vi "Files.Get Result Dir List from Root Dir.vi"(10 "SN Len":i32=10, 11 "RootDir":path) -> (2 "Cnt":i32, 3 "Result Dirs":path[](array[path]))   [LabVIEW 2024]
panel:
  # "Result = SN_Date_Time. . . .\nEX: FB94414A63_20191118_103814"
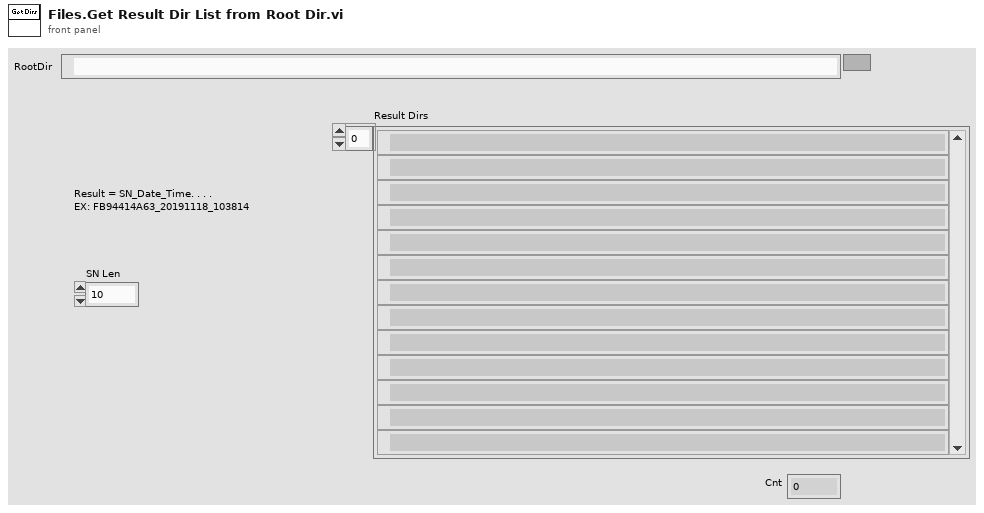
[diagram p1: front panel]
types:
  T1 = cluster{"RsltDirs":path[], "RootDir":path, "RootName":string}
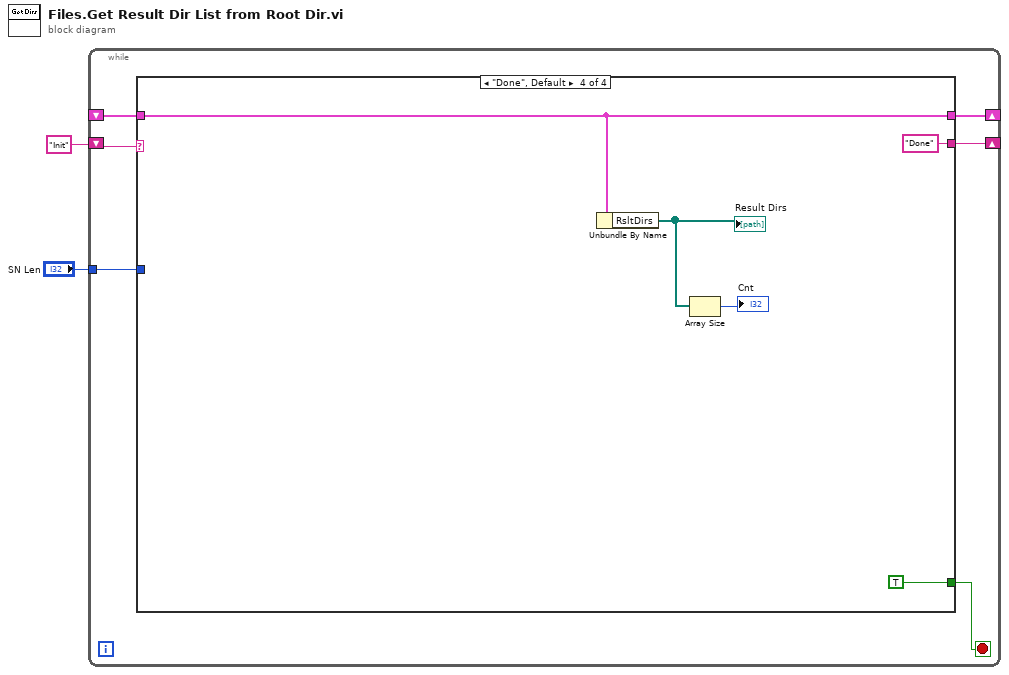
[diagram p0: block diagram]
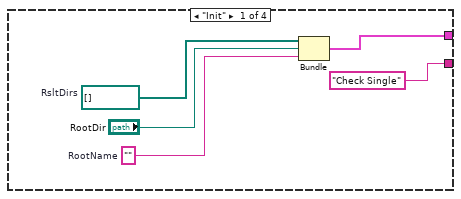
[diagram p2: hidden frame]
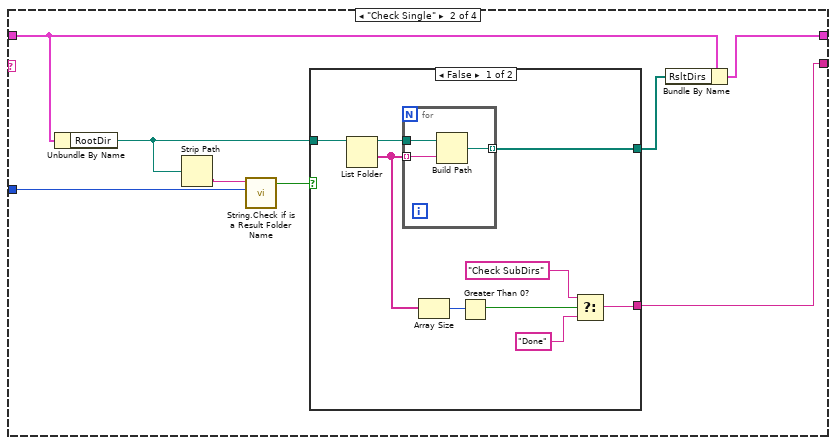
[diagram p3: hidden frame]
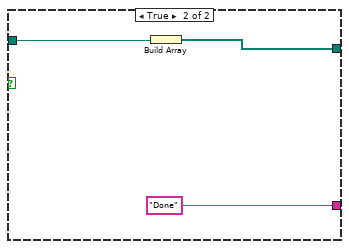
[diagram p4: hidden frame]
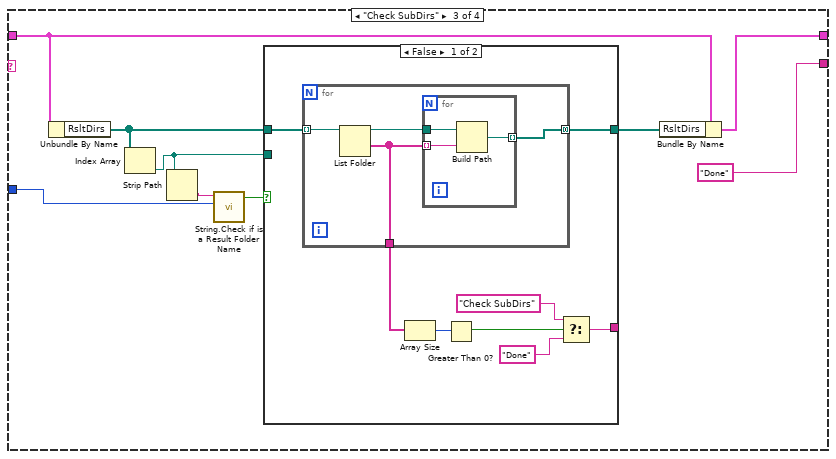
[diagram p5: hidden frame]
diagram:
  n1 = while {
    shift-right: [w6] -> _
    shift-left: _ -> [w7]
    shift-right: [w5] -> _
    shift-left: "Init" -> [w8]
    tunnel: "SN Len" -> [w3]
    stop <- w4 stop-if-true
    n2 = case shown="\"Done\", Default" w8 {
      tunnel: w7 -> [_ w20 w44 w64]
      tunnel: [w12 w21 w45 w64] -> w6
      tunnel: ["Check Single" w15 "Done" "Done"] -> w5
      tunnel: [_ _ _ TRUE] -> w4
      tunnel: w3 -> [_ w18 w40 _]
      frame "Init" {
        w10 = ""  # RootName
        w13 = path[] []  # RsltDirs
        n3 = Bundle("RsltDirs"=w13, "RootDir"="RootDir", "RootName"=w10) -> (w12:T1)  [unwired: 1 in]
      }
      frame "Check Single" {
        n4 = Unbundle By Name(w20) -> ("RootDir"=w16:path)
        n5 = Strip Path(path=w16) -> (name=w19:string)  [unwired: 1 out]
        n6 = call "String.Check if is a Result Folder Name.vi"("SN Len"=w18, "Name"=w19) -> ("OK"=w17:bool)  [unwired: 5 in, 4 out]
        n7 = case shown="False" w17 {
          tunnel: w16 -> [w30 w35]
          tunnel: [w22 "Done"] -> w15
          tunnel: [w28 w34] -> w14
          frame False {
            n8 = List Folder(path=w30) -> (path out=w29:path, folder names=w27:string[])  [unwired: 3 in, 2 out]
            n9 = for {
              tunnel: w29 -> [w33]
              tunnel: w27 -> [w32] mode=indexing
              tunnel: [w31] -> w28 mode=indexing
              n10 = Build Path(base path=w33, name or relative path=w32) -> (appended path=w31:path)
            }
            n11 = Array Size(array=w27) -> (size(s)=w26:i32)
            n12 = Greater Than 0?(x=w26) -> (x > 0?=w24:bool)
            n13 = Select(t="Check SubDirs", s=w24, f="Done") -> (s? t:f=w22:string)
          }
          frame True {
            n14 = Build Array(w35) -> (w34:path[])
          }
        }
        n15 = Bundle By Name(cluster=w20, "RsltDirs"=w14) -> (w21:T1)
      }
      frame "Check SubDirs" {
        n16 = Unbundle By Name(w44) -> ("RsltDirs"=w39:path[])
        n17 = Index Array(array=w39) -> (element=w41:path)  [unwired: 1 in]
        n18 = Strip Path(path=w41) -> (name=w43:string)  [unwired: 1 out]
        n19 = call "String.Check if is a Result Folder Name.vi"("SN Len"=w40, "Name"=w43) -> ("OK"=w42:bool)  [unwired: 5 in, 4 out]
        n20 = case shown="False" w42 {
          tunnel: w41 -> [_ _]
          tunnel: w39 -> [w53 w61]
          tunnel: [w52 w61] -> w38
          tunnel: [w46 _] -> _
          frame False {
            n21 = for {
              tunnel: w53 -> [w56] mode=indexing
              tunnel: [w55] -> w52 mode=concatenating
              tunnel: [w54] -> w47
              n22 = List Folder(path=w56) -> (path out=w57:path, folder names=w54:string[])  [unwired: 3 in, 2 out]
              n23 = for {
                tunnel: w57 -> [w60]
                tunnel: w54 -> [w59] mode=indexing
                tunnel: [w58] -> w55 mode=indexing
                n24 = Build Path(base path=w60, name or relative path=w59) -> (appended path=w58:path)
              }
            }
            n25 = Array Size(array=w47) -> (size(s)=w51:i32)
            n26 = Greater Than 0?(x=w51) -> (x > 0?=w49:bool)
            n27 = Select(t="Check SubDirs", s=w49, f="Done") -> (s? t:f=w46:string)
          }
          frame True {
          }
        }
        n28 = Bundle By Name(cluster=w44, "RsltDirs"=w38) -> (w45:T1)
      }
      frame "Done", Default {
        n29 = Unbundle By Name(w64) -> ("RsltDirs"=w62:path[])
        "Result Dirs" <- w62
        n30 = Array Size(array=w62) -> (size(s)=→"Cnt":i32)
      }
    }
  }
